vi "power value.vi"(6 "label":T1, 8 "error in (no error)":errorcluster, 10 "B":refnum<class "Value.lvclass">, 11 "A":refnum<class "Value.lvclass">) -> (0 "error out":errorcluster, 2 "C":refnum<class "Value.lvclass">, 3 "A out":refnum<class "Value.lvclass">)   [LabVIEW 2023, in "LabGRAD.lvlib" / "Value.lvclass"]
uses:
  Value.lvclass
  operation.ctl
  Value.lvclass/Value.ctl
  UiObjects/string control.ctl
  UiObjects/UiObjects.lvclass
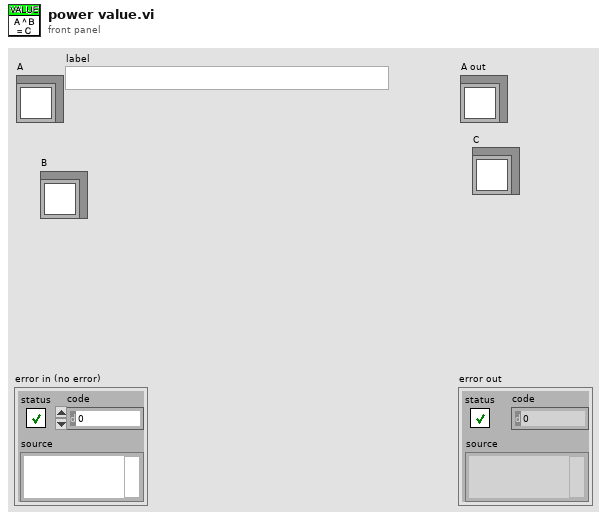
[diagram p1: front panel]
types:
  T1 = typedef "UiObjects.lvlib/UiObjects.lvclass/string control.ctl" = string
  T2 = typedef "LabGRAD.lvlib/Value.lvclass/operation.ctl" = enum16{"nop", "add", "subtract", "power", "multiply", "divide"}
  T3 = typedef "UiObjects.lvlib/UiObjects.lvclass/numeric value control.ctl" = dbl
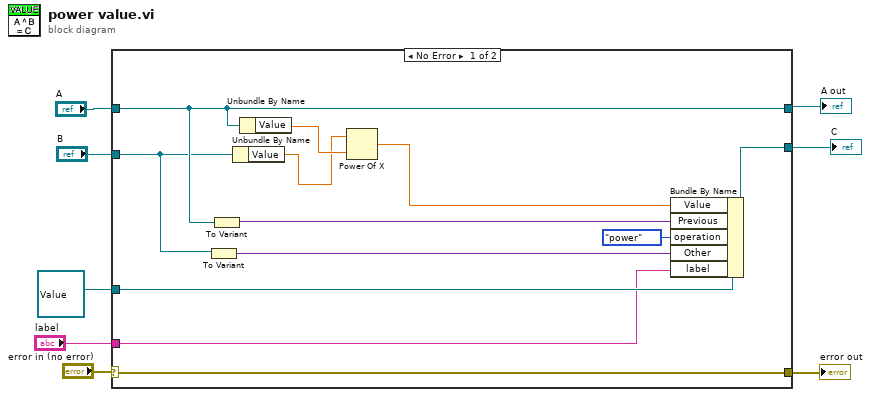
[diagram p0: block diagram]
diagram:
  n1 = case shown="No Error" "error in (no error)" {
    selector: "error in (no error)" -> [w20 w23]
    tunnel: [w20 w23] -> w6
    tunnel: [w19 w22] -> w7
    tunnel: "A" -> [w19 w22]
    tunnel: [w18 w21] -> w3
    tunnel: refnum<class "Value.lvclass"> refnum ("B") -> [w17 w21]
    tunnel: "B" -> [w13 _]
    tunnel: "label" -> [w9 _]
    frame No Error {
      n2 = To Variant(anything=w13) -> (Variant=w15:variant)
      n3 = To Variant(anything=w19) -> (Variant=w14:variant)
      n4 = Unbundle By Name(w13) -> ("Value"=w11:T3)
      n5 = Unbundle By Name(w19) -> ("Value"=w12:T3)
      n6 = Power Of X(1:w12, 2:w11) -> (0:w10:T3)
      n7 = Bundle By Name(cluster=w17, "Value"=w10, "Previous"=w14, "operation"=operation."power", "Other"=w15, "label"=w9) -> (w18:refnum<class "Value.lvclass">)
    }
    frame Error {
    }
  }
  "error out" <- w6
  "A out" <- w7
  "C" <- w3
